vi "Database Connection.vi"(8 "error in (no error)":errorcluster) -> (0 "error out":errorcluster)   [LabVIEW 2013]
uses:
  <userlib>/Accelerator/User Interface/Controls/Post_Dust_Event.ctl
  <userlib>/Accelerator/User Interface/Controls/File_location.ctl
  <userlib>/Accelerator/User Interface/Controls/DisplayExperimentSetting.ctl
  <userlib>/Accelerator/User Interface/Controls/Dust_Properties.ctl
  <userlib>/Accelerator/User Interface/Controls/source_builders.ctl
  <userlib>/Accelerator/User Interface/Controls/Operator.ctl
  <userlib>/Accelerator/User Interface/Controls/dust_type_indicator.ctl
  <userlib>/Accelerator/User Interface/Controls/Post_Dust_Event_small.ctl
  <vilib>/Utility/miscctls.llb/LVPointTypeDef.ctl
  <userlib>/Accelerator/User Interface/Controls/Dust_Event.ctl
  <userlib>/Accelerator/User Interface/Controls/Signal.ctl
  <userlib>/Accelerator/User Interface/Controls/Role ID.ctl
  <userlib>/Accelerator/User Interface/Controls/Hardware ID.ctl
  <userlib>/Accelerator/User Interface/Controls/Estimate_source.ctl
  <userlib>/Accelerator/Global Variables/Action Items.ctl
  <userlib>/Accelerator/Global Variables/throttle.vi
  <userlib>/Accelerator/Sub-Polymorphic/post_dust_event_small.vi
  <userlib>/Accelerator/Sub-Polymorphic/post_dust_event_big.vi
panel:
  in  "Tab Control":enum32{"Status", "Processing", "Error Handling"}(tab)
  out "Small?":bool
  out "Dust Properties":T1
  in  "Update dust info":bool
  in  "Update Experiment Settings":bool
  out "output cluster":T2={"Current Experiment Name:"="NDA", "Current Experiment Description:"="Database testing during NDA run in August.", "Current Experiment Group ID:"="Database Testing", "Experiment Settings Last Updated At:"=timestamp(3427974586.5021 s since 1904-01-01)}
  out "Dust Type":T3 {"Batch" step=1; "Type" step=1; "Dust Source Builder:" items=["Keith Drake", "Nick Beaty", "Anthony Shu", "David James", "John Fontanese"]}
  in  "Update Operator":bool
  out "Current Operator:":T5 {"Operator" items=["Giraffe", "Andrew Collette", "Keith Drake", "Anthony Shu", "Evan Thomas", "Nicholaus Beaty", "David James", "John Fontanese", ""]}
  out "# Events posted during current session:":i32=96
  out "# Events in dust event queue:":i32=388
  out "Dust Event Processing Big":T6={"Dust Event ID"=0, "Integer Timestamp"=13461087072182, "Velocity"=nan, "Mass"=nan, "Charge"=2.2111935e-15, "Radius"=0.0, "Experiment Settings"=0.0, "Pelletron ID"=0, "Estimate Quality"=0.0, "File Location"=0, "id_dust_info"=0.0, "DCS 1 X"=0.0, "DCS 1 Y"=0.0, "DCS 2 X"=0.0, "DCS 2 Y"=0.0} {"File Location" items=["Unknown"=-1, "Storage"=0, "Processing"=1, "Unmerged"=2]}
  out "Dust Event Processing Small":T8 {"File Location" items=["Unknown"=-1, "Storage"=0, "Processing"=1, "Unmerged"=2]}
  in  "Write Signals":bool=TRUE
  out "Test":bool caption="Test Database in use:"
  out "Test 2":bool=TRUE caption="Production Database in use:"
  in  "Clear Errors":bool
  in  "Exit":bool=TRUE
  # "Database Connection V3"
  # "Experiment Status:"
  # "Dust Information"
  # "Dust Event"
  # "Dust Event Small"
  # "ODBC Connection Status:"
  # "Error Status:"
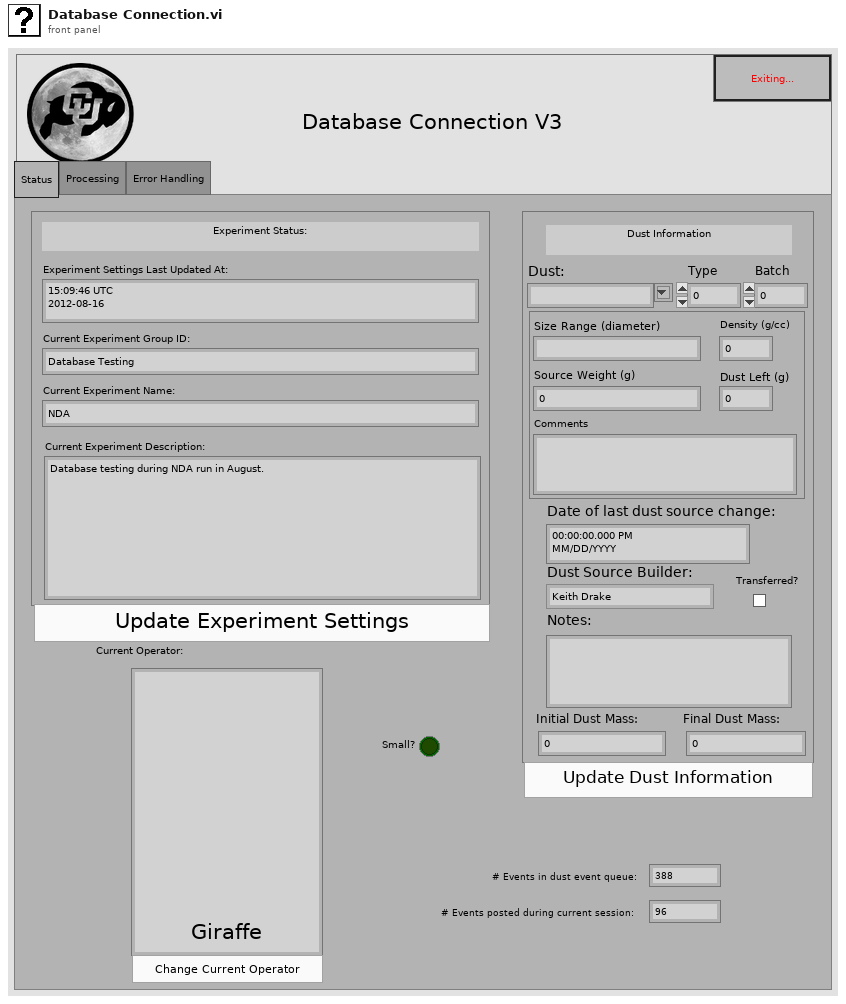
[diagram p1: front panel]
types:
  T1 = typedef "dust_type_indicator.ctl" = cluster{"id_dust_type":i32, "Size Range (diameter)":string, "Density (g/cc)":dbl, "Source Weight (g)":dbl, "Dust Left (g)":dbl, "Comments":string}
  T2 = typedef "DisplayExperimentSetting.ctl" = cluster{"Current Experiment Name:":string, "Current Experiment Description:":string, "Current Experiment Group ID:":string, "Experiment Settings Last Updated At:":timestamp}
  T3 = typedef "Dust_Properties.ctl" = cluster{"Dust info id":u16, "Integer Timestamp":i64, "Dust:":string, "Dust Source Builder:":T4, "Notes:":string, "Date of last dust source change:":timestamp, "Initial Dust Mass:":dbl, "Final Dust Mass:":dbl, "Type":u16, "Batch":u16, "dust type id":u16, "Transferred?":bool}
  T4 = typedef "source_builders.ctl" = u16
  T5 = typedef "Operator.ctl" = cluster{"Timestamp":i64, "Operator":u16}
  T6 = typedef "Post_Dust_Event.ctl" = cluster{"Dust Event ID":i64, "Integer Timestamp":i64, "Velocity":sgl, "Mass":sgl, "Charge":sgl, "Radius":sgl, "Experiment Settings":dbl, "Pelletron ID":i32, "Estimate Quality":sgl, "File Location":T7, "id_dust_info":dbl, "DCS 1 X":sgl, "DCS 1 Y":sgl, "DCS 2 X":sgl, "DCS 2 Y":sgl}
  T7 = typedef "File_location.ctl" = i8
  T8 = typedef "Post_Dust_Event_small.ctl" = cluster{"Dust Event ID":i64, "Integer Timestamp":i64, "Velocity":sgl, "Mass":sgl, "Charge":sgl, "Radius":sgl, "Needle Voltage (MV)":dbl, "Experiment Settings":dbl, "Estimate Quality":sgl, "File Location":T7, "id_dust_info":dbl}
  T9 = typedef "LVPointTypeDef.ctl" = cluster{"Horizontal":i16, "Vertical":i16}
  T10 = typedef "Dust_Event.ctl" = cluster{"Time Stamp":timestamp, "Velocity":sgl, "Mass":sgl, "Charge":sgl, "Radius":sgl, "Array":T11[], "Dust Event ID":i64, "Passed_3rd_Detector":bool, "Estimate Source":T14, "Estimate Quality":sgl}
  T11 = typedef "Signal.ctl" = cluster{"Signal ID":i64, "Time Stamp":timestamp, "Dust Event ID":i64, "Role ID":T12, "Data":sgl[], "Signal Length":i32, "dt":sgl, "Offset":dbl, "Hardware ID":T13}
  T12 = typedef "Role ID.ctl" = enum16{"First_Detector", "Second_Detector", "Third_Detector", "LeCroy_CH1", "LeCroy_CH2", "LeCroy_CH3", "LeCroy_CH4", "PSU", "DCS 1", "DCS 2"}
  T13 = typedef "Hardware ID.ctl" = enum16{"Unknown", "CSA 1", "CSA 2", "CSA 3", "CSA 4", "CSA 5", "CSA 6", "DCS 1", "DCS 2"}
  T14 = typedef "Estimate_source.ctl" = i8
  T15 = typedef "Action Items.ctl" = enum16{"Initialize", "Get", "Set"}
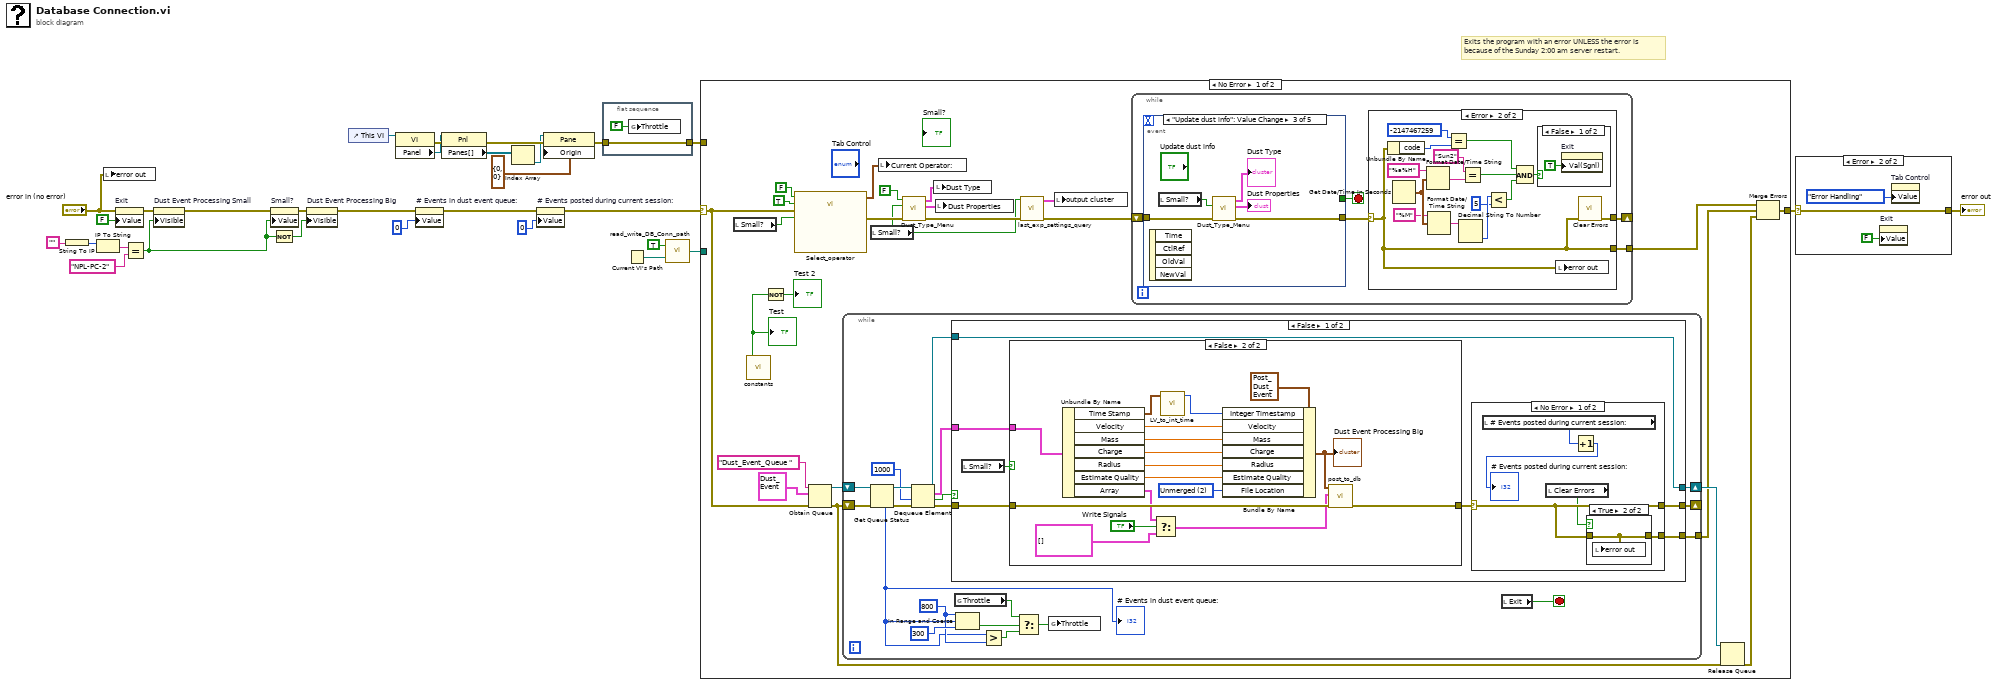
[diagram p0: block diagram]
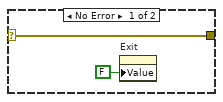
[diagram p2: hidden frame]
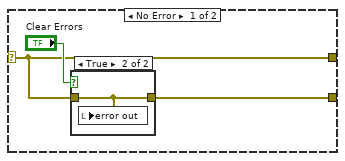
[diagram p3: hidden frame]
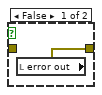
[diagram p4: hidden frame]
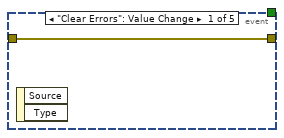
[diagram p6: hidden frame]
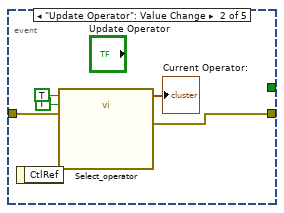
[diagram p7: hidden frame]
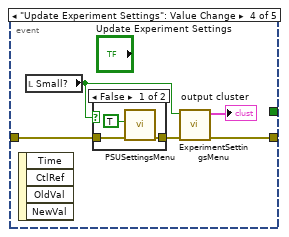
[diagram p8: hidden frame]
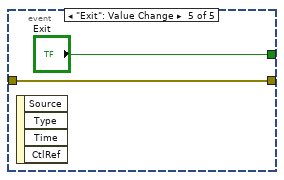
[diagram p10: hidden frame]
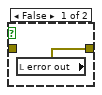
[diagram p11: hidden frame]
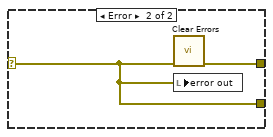
[diagram p12: hidden frame]
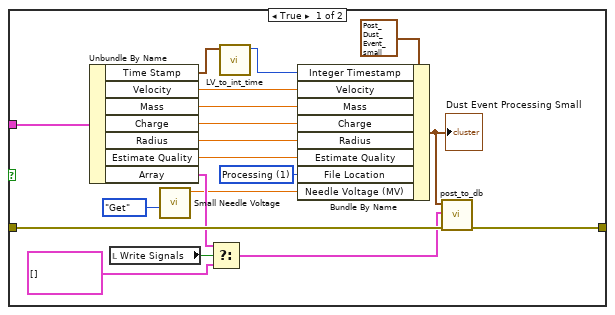
[diagram p13: hidden frame]
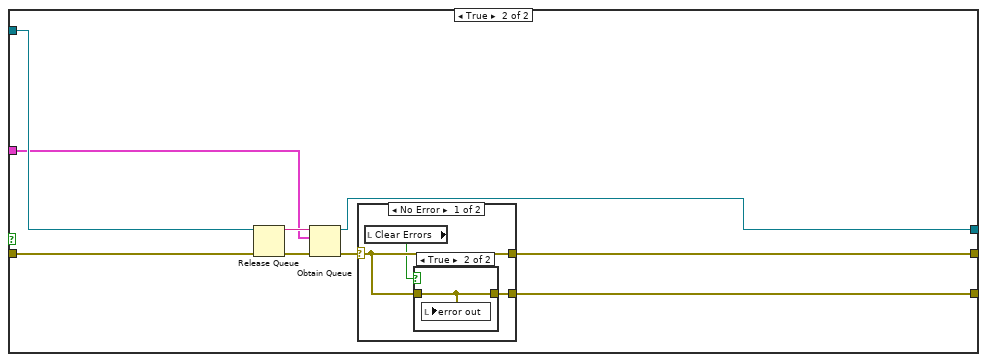
[diagram p14: hidden frame]
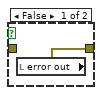
[diagram p15: hidden frame]
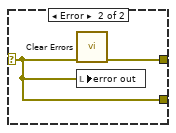
[diagram p16: hidden frame]
diagram:
  # "Exits the program with an error UNLESS the error is\nbecause of the Sunday 2:00 am server restart."
  n1 = String To IP(1:"") -> (0:w18:u32)
  n2 = IP To String(2:w18) -> (0:w17:string)  [unwired: 1 in]
  n3 = local write "error out"("error in (no error)") -> ()
  n4 = property on="Exit" class="Bool (strict)"(error in="error in (no error)", "Value"=FALSE ("Exit")) -> (error out=w23:errorcluster)  [unwired: 1 in, 1 out]
  n5 = Equal?(x=w17, y="NPL-PC-2") -> (x = y?=w13:bool)
  n6 = property on="Dust Event Processing Small" class="Clust (strict)"(error in=w23, "Visible"=w13) -> (error out=w12:errorcluster)  [unwired: 1 in, 1 out]
  n7 = property on="Small?" class="Bool (strict)"(error in=w12, "Value"=w13) -> (error out=w2:errorcluster)  [unwired: 1 in, 1 out]
  n8 = Not(x=w13) -> (.not. x?=w3:bool)
  n9 = property on="Dust Event Processing Big" class="Clust (strict)"(error in=w2, "Visible"=w3) -> (error out=w1:errorcluster)  [unwired: 1 in, 1 out]
  n10 = control-ref of="This VI"() -> (w30:refnum<vi>)
  n11 = property class="VI"(reference=w30) -> (error out=w29:errorcluster, "Panel"=w28:refnum<vi>)  [unwired: 1 in, 1 out]
  n12 = property on="# Events in dust event queue:" class="DigNum (strict)"(error in=w1, "Value"=0 ("# Events in dust event queue:")) -> (error out=w9:errorcluster)  [unwired: 1 in, 1 out]
  n13 = property class="Pnl"(reference=w28, error in=w29) -> (error out=w27:errorcluster, "Panes[]"=w26:refnum<vi>[])  [unwired: 1 out]
  n14 = Index Array(array=w26) -> (element=w25:refnum<vi>)  [unwired: 1 in]
  n15 = property on="# Events posted during current session:" class="DigNum (strict)"(error in=w9, "Value"=0 ("# Events in dust event queue:")) -> (error out=w8:errorcluster)  [unwired: 1 in, 1 out]
  n16 = property class="Pane"(reference=w25, error in=w27, "Origin"=T9 {"Horizontal"=0, "Vertical"=0}) -> (error out=w20:errorcluster)  [unwired: 1 out]
  n17 = flat-sequence {
    tunnel: [w32] -> w21
    tunnel: w20 -> [w32]
    frame #0 {
      n18 = global write "throttle.vi" "Throttle"(FALSE ("Throttle")) -> ()
    }
  }
  n19 = Current VI's Path() -> (path=w5:path)
  n20 = call <userlib>:"read_write_DB_Conn_path.vi"("DB Connection Path in"=w5, "Write?"=TRUE) -> ("DB Connection Path"=w4:path)
  n21 = case shown="No Error" w8 {
    selector: w8 -> [w34 w194]
    tunnel: [w39 w194] -> w15
    tunnel: w21 -> [_ _]
    tunnel: w4 -> [_ _]
    frame No Error {
      n22 = local read "Small?"() -> (w46:bool)
      n23 = call <userlib>:"constants.vi"() -> ("Testing"=w33:bool)  [unwired: 3 out]
      "Test" <- w33
      n24 = Not(x=w33) -> (.not. x?=→"Test 2":bool)
      n25 = call <userlib>:"Select_operator.vi"("Enable"=FALSE, "sub vi?"=TRUE, "error in (no error)"=w34, "small?"=w46) -> ("Operator Cluster 2"=w49:T5, "error out"=w44:errorcluster)  [unwired: 13 in, 1 out]
      n26 = Obtain Queue(name (unnamed)="Dust_Event_Queue ", element data type=T10 {"Time Stamp"=timestamp(0 s since 1904-01-01), "Velocity"=0.0, "Mass"=0.0, "Charge"=0.0, "Radius"=0.0, "Array"=[], "Dust Event ID"=0, "Passed_3rd_Detector"=FALSE, "Estimate Source"=0, "Estimate Quality"=0.0} ("Cluster"), error in (no error)=w34) -> (queue out=w53:refnum<queue>, error out=w55:errorcluster)  [unwired: 2 in, 1 out]
      n27 = while {
        shift-right: [w109] -> _
        shift-left: w55 -> [w124]
        shift-right: [w123] -> w54
        shift-left: w53 -> [w125]
        tunnel: [w107] -> w45
        stop <- w108 stop-if-true
        w114 = 800 ("y")
        n28 = Get Queue Status(queue=w125, error in (no error)=w124) -> (queue out=w121:refnum<queue>, error out=w119:errorcluster, # elements in queue=w106:i32)  [unwired: 1 in, 5 out]
        "# Events in dust event queue:" <- w106
        n29 = Dequeue Element(queue=w121, timeout in ms (-1)=u32 1000 ("milliseconds to wait"), error in (no error)=w119) -> (queue out=w120:refnum<queue>, element=w122:T10, timed out?=w117:bool, error out=w118:errorcluster)
        n30 = case shown="False" w117 {
          tunnel: w120 -> [w132 w186]
          tunnel: w118 -> [w130 w178]
          tunnel: [w132 w184] -> w123
          tunnel: [w127 w180] -> w109
          tunnel: w122 -> [w131 w182]
          tunnel: [w126 w179] -> w107
          frame False {
            n31 = local read "Small?"() -> (w129:bool)
            n32 = case shown="False" w129 {
              tunnel: w131 -> [w152 w169]
              tunnel: w130 -> [w151 w168]
              tunnel: [w150 w167] -> w128
              frame True {
                w147 = T7 1 items=["Unknown"=-1, "Storage"=0, "Processing"=1, "Unmerged"=2] ("File Location")
                n33 = Unbundle By Name(w152) -> ("Time Stamp"=w159:timestamp, "Velocity"=w155:sgl, "Mass"=w156:sgl, "Charge"=w157:sgl, "Radius"=w158:sgl, "Estimate Quality"=w146:sgl, "Array"=w145:T11[])
                n34 = local read "Write Signals"() -> (w144:bool)
                n35 = call <userlib>:"Small Needle Voltage.vi"("Action"=Action_Items."Get") -> ("Output Pelletron Voltage"=w142:dbl)  [unwired: 10 in]
                n36 = Select(t=w145, s=w144, f=T11[] []) -> (s? t:f=w148:T11[])
                n37 = call <userlib>:"LV_to_int_time.vi"("Time Stamp"=w159) -> ("Integer Time"=w160:i64)  [unwired: 8 in, 1 out]
                n38 = Bundle By Name(cluster=T8 {"Dust Event ID"=0, "Integer Timestamp"=0, "Velocity"=0.0, "Mass"=0.0, "Charge"=0.0, "Radius"=0.0, "Needle Voltage (MV)"=0.0, "Experiment Settings"=0.0, "Estimate Quality"=0.0, "File Location"=0, "id_dust_info"=0.0} ("Cluster"), "Integer Timestamp"=w160, "Velocity"=w155, "Mass"=w156, "Charge"=w157, "Radius"=w158, "Estimate Quality"=w146, "File Location"=w147, "Needle Voltage (MV)"=w142) -> (w153:T8)
                "Dust Event Processing Small" <- w153
                n39 = call-poly <userlib>:"post_to_db.vi"("error in (no error)"=w151, "Signal Array"=w148, "Cluster"=w153) -> ("error out"=w150:errorcluster)  [unwired: 6 in, 2 out]
              }
              frame False {
                w163 = T7 2 items=["Unknown"=-1, "Storage"=0, "Processing"=1, "Unmerged"=2] ("File Location")
                n40 = Unbundle By Name(w169) -> ("Time Stamp"=w176:timestamp, "Velocity"=w172:sgl, "Mass"=w173:sgl, "Charge"=w174:sgl, "Radius"=w175:sgl, "Estimate Quality"=w162:sgl, "Array"=w161:T11[])
                n41 = Select(t=w161, s="Write Signals", f=T11[] []) -> (s? t:f=w164:T11[])
                n42 = call <userlib>:"LV_to_int_time.vi"("Time Stamp"=w176) -> ("Integer Time"=w177:i64)  [unwired: 8 in, 1 out]
                n43 = Bundle By Name(cluster=T6 {"Dust Event ID"=0, "Integer Timestamp"=0, "Velocity"=0.0, "Mass"=0.0, "Charge"=0.0, "Radius"=0.0, "Experiment Settings"=0.0, "Pelletron ID"=0, "Estimate Quality"=0.0, "File Location"=0, "id_dust_info"=0.0, "DCS 1 X"=0.0, "DCS 1 Y"=0.0, "DCS 2 X"=0.0, "DCS 2 Y"=0.0} ("Cluster 2"), "Integer Timestamp"=w177, "Velocity"=w172, "Mass"=w173, "Charge"=w174, "Radius"=w175, "Estimate Quality"=w162, "File Location"=w163) -> (w170:T6)
                "Dust Event Processing Big" <- w170
                n44 = call-poly <userlib>:"post_to_db.vi"("error in (no error)"=w168, "Signal Array"=w164, "Cluster"=w170) -> ("error out"=w167:errorcluster)  [unwired: 6 in, 2 out]
              }
            }
            n45 = case shown="No Error" w128 {
              selector: w128 -> [w137 w140]
              tunnel: [w137 w141] -> w127
              tunnel: [w136 w140] -> w126
              frame No Error {
                n46 = local read "# Events posted during current session:"() -> (w134:i32)
                n47 = local read "Clear Errors"() -> (w135:bool)
                n48 = Increment(x=w134) -> (x+1=→"# Events posted during current session:":i32)
                n49 = case shown="True" w135 {
                  tunnel: w137 -> [_ w139]
                  tunnel: [w138 w139] -> w136
                  frame False {
                    n50 = local read "error out"() -> (w138:errorcluster)
                  }
                  frame True {
                    n51 = local write "error out"(w139) -> ()
                  }
                }
              }
              frame Error {
                n52 = call <vilib>:"Clear Errors.vi"("error in (no error)"=w140) -> ("error out"=w141:errorcluster)  [unwired: 6 in]
                n53 = local write "error out"(w140) -> ()
              }
            }
          }
          frame True {
            n54 = Release Queue(queue=w186, error in (no error)=w178) -> (queue name=w183:string, error out=w185:errorcluster)  [unwired: 1 in, 1 out]
            n55 = Obtain Queue(name (unnamed)=w183, element data type=w182, error in (no error)=w185) -> (queue out=w184:refnum<queue>, error out=w181:errorcluster)  [unwired: 2 in, 1 out]
            n56 = case shown="No Error" w181 {
              selector: w181 -> [w189 w192]
              tunnel: [w189 w193] -> w180
              tunnel: [w188 w192] -> w179
              frame No Error {
                n57 = local read "Clear Errors"() -> (w187:bool)
                n58 = case shown="True" w187 {
                  tunnel: w189 -> [_ w191]
                  tunnel: [w190 w191] -> w188
                  frame False {
                    n59 = local read "error out"() -> (w190:errorcluster)
                  }
                  frame True {
                    n60 = local write "error out"(w191) -> ()
                  }
                }
              }
              frame Error {
                n61 = call <vilib>:"Clear Errors.vi"("error in (no error)"=w192) -> ("error out"=w193:errorcluster)  [unwired: 6 in]
                n62 = local write "error out"(w192) -> ()
              }
            }
          }
        }
        n63 = global read "throttle.vi" "Throttle"() -> (w110:bool)
        n64 = In Range and Coerce(upper limit=w114, x=w106, lower limit=300) -> (In Range?=w113:bool)  [unwired: 1 out]
        n65 = Greater?(x=w106, y=w114) -> (0:w112:bool)
        n66 = Select(t=w110, s=w113, f=w112) -> (s? t:f=w111:bool)
        n67 = global write "throttle.vi" "Throttle"(w111) -> ()
        n68 = local read "Exit"() -> (w108:bool)
      }
      n69 = local read "Small?"() -> (w35:bool)
      n70 = local write "Current Operator:"(w49) -> ()
      n71 = call <userlib>:"Dust_Type_Menu.vi"("error in (no error)"=w44, "Small?"=w35, "Enable"=FALSE) -> ("error out"=w38:errorcluster, "Dust Properties"=w42:T1, "Dust Info"=w43:T3)  [unwired: 5 in, 1 out]
      n72 = local write "Dust Type"(w43) -> ()
      n73 = local write "Dust Properties"(w42) -> ()
      n74 = call <userlib>:"last_exp_settings_query.vi"("error in (no error)"=w38, "Small?"=w35) -> ("error out"=w36:errorcluster, "Experiment Settings"=w37:T2)  [unwired: 4 in, 4 out]
      n75 = local write "output cluster"(w37) -> ()
      n76 = while {
        shift-right: [w59] -> _
        shift-left: w36 -> [w57]
        tunnel: [w58] -> w40
        stop <- w61 stop-if-true
        n77 = event shown="[2] \"Update dust info\": Value Change" {
          selector: _ -> [_ _ _ _ _]
          dyn-events: _ -> [_ _ _ _ _]
          timeout: _ -> [_ _ _ _ _]
          tunnel: w57 -> [w84 w89 w92 w97 w104]
          tunnel: [w84 w86 w93 w96 w104] -> w60
          tunnel: [_ _ _ _ "Exit"] -> w61
          event "Clear Errors": Value Change {
            n78 = event-data() -> ()  [unwired: 1 in, 2 out]
          }
          event "Update Operator": Value Change {
            n79 = event-data() -> ()  [unwired: 1 in, 1 out]
            n80 = call <userlib>:"Select_operator.vi"("Enable"=TRUE, "sub vi?"=TRUE, "error in (no error)"=w89) -> ("Operator Cluster 2"=→"Current Operator:":T5, "error out"=w86:errorcluster)  [unwired: 14 in, 1 out]
          }
          event "Update dust info": Value Change {
            n81 = event-data() -> ()  [unwired: 1 in, 4 out]
            n82 = local read "Small?"() -> (w90:bool)
            n83 = call <userlib>:"Dust_Type_Menu.vi"("error in (no error)"=w92, "Small?"=w90) -> ("error out"=w93:errorcluster, "Dust Properties"=→"Dust Properties":T1, "Dust Info"=→"Dust Type":T3)  [unwired: 6 in, 1 out]
          }
          event "Update Experiment Settings": Value Change {
            n84 = event-data() -> ()  [unwired: 1 in, 4 out]
            n85 = local read "Small?"() -> (w98:bool)
            n86 = case shown="False" w98 {
              tunnel: w97 -> [w102 w103]
              tunnel: [w100 w103] -> w99
              frame False {
                n87 = call <userlib>:"PSUSettingsMenu.vi"("error in (no error)"=w102, "sub vi?"=TRUE) -> ("error out"=w100:errorcluster)  [unwired: 7 in, 2 out]
              }
              frame True {
              }
            }
            n88 = call <userlib>:"ExperimentSettingsMenu.vi"("error in (no error)"=w99, "Small?"=w98) -> ("error out"=w96:errorcluster, "output cluster"=→"output cluster":T2)  [unwired: 8 in]
          }
          event "Exit": Value Change {
            n89 = event-data() -> ()  [unwired: 1 in, 4 out]
          }
        }
        n90 = case shown="Error" w60 {
          selector: w60 -> [w63 w78]
          tunnel: [w63 w82] -> w59
          tunnel: [w62 w78] -> w58
          frame No Error {
            n91 = case shown="True" "Clear Errors" {
              tunnel: w63 -> [_ w66]
              tunnel: [w65 w66] -> w62
              frame False {
                n92 = local read "error out"() -> (w65:errorcluster)
              }
              frame True {
                n93 = local write "error out"(w66) -> ()
              }
            }
          }
          frame Error {
            n94 = Unbundle By Name(w78) -> ("code"=w80:i32)
            n95 = Get Date/Time In Seconds() -> (seconds since 1Jan1904=w75:timestamp)
            n96 = Format Date/Time String(time format string (%c)="%a%H", seconds (now)=w75) -> (date/time string=w76:string)  [unwired: 1 in]
            n97 = Format Date/Time String(time format string (%c)="%M", seconds (now)=w75) -> (date/time string=w73:string)  [unwired: 1 in]
            n98 = Equal?(x=-2147467259 ("y"), y=w80) -> (x = y?=w70:bool)
            n99 = Decimal String To Number(string=w73) -> (number=w72:i32)  [unwired: 2 in, 1 out]
            n100 = Equal?(x="Sun2", y=w76) -> (x = y?=w69:bool)
            n101 = Less?(x=w72, y=5) -> (x < y?=w68:bool)
            n102 = Compound Arithmetic op=AND(w70, w69, w68) -> (w67:bool)
            n103 = case shown="False" w67 {
              frame False {
                n104 = property on="Exit" class="Bool (strict)"("Val(Sgnl)"=TRUE ("Value (Signaling)")) -> ()  [unwired: 2 in, 2 out]
              }
              frame True {
              }
            }
            n105 = local write "error out"(w78) -> ()
            n106 = call <vilib>:"Clear Errors.vi"("error in (no error)"=w78) -> ("error out"=w82:errorcluster)  [unwired: 6 in]
          }
        }
      }
      n107 = Release Queue(queue=w54, error in (no error)=w55) -> (error out=w47:errorcluster)  [unwired: 1 in, 2 out]
      n108 = Merge Errors(w40, w45, w47) -> (w39:errorcluster)
    }
    frame Error {
    }
  }
  n109 = case shown="Error" w15 {
    selector: w15 -> [w196 w199]
    tunnel: [w196 w199] -> w14
    frame No Error {
      n110 = property on="Exit" class="Bool (strict)"("Value"=FALSE ("Exit")) -> ()  [unwired: 2 in, 2 out]
    }
    frame Error {
      n111 = property on="Exit" class="Bool (strict)"("Value"=FALSE ("Exit")) -> ()  [unwired: 2 in, 2 out]
      n112 = property on="Tab Control" class="TabCtl (strict)"("Value"=enum32{"Status", "Processing", "Error Handling"}."Error Handling" ("Tab Control")) -> ()  [unwired: 2 in, 2 out]
    }
  }
  "error out" <- w14
